vi "Barrier for IV curve.vi"() -> ()   [LabVIEW 2016]
panel:
  out "Barrier average 2":dbl=0.21135603486952198 format="%#_6p"
  out "Barrier for backward IV 2":dbl=0.22242669607101634 format="%#_6p"
  out "Barrier for forward IV 2":dbl=0.20028537366802762 format="%#_6p"
  out "IV after extracting current offset at zero bias":cluster{"Time Stamps":dbl[], dbl[]}[](graph)
  out "IV after extracting current offset at zero bias":cluster{"Time Stamps":dbl[], "Y":dbl[]}(graph)
  out "Backward offset":dbl=1.766897762857724e-08 format="%#_6p"
  out "Forward offset":dbl=-1.6472324480187406e-08 format="%#_6p"
  out "size(s)":i32=525
  out "IV without extracting current offset at zero bias":cluster{"Time Stamps":dbl[], "Y":dbl[]}[](graph)
  out "Barrier average":dbl=0.28652409507268245 format="%#_6p"
  out "Barrier for forward IV":dbl=0.24381885922702945 format="%#_6p"
  out "Barrier for backward IV":dbl=0.32922933091833545 format="%#_6p"
  in  "Linear fitting step":i32=32
  out "min index(es)":i32=394 format="%.0p"
  out "min value":dbl=-0.49999890379533224 format="%#_6p"
  out "max index(es)":i32=131 format="%.0p"
  out "max value":dbl=0.49999729304706686 format="%#_6p"
  in  "Input IV curve":cluster{"Time Stamps":dbl[], "Y":dbl[]}(graph)={"Time Stamps"=array[525 elements], "Y"=array[525 elements]}
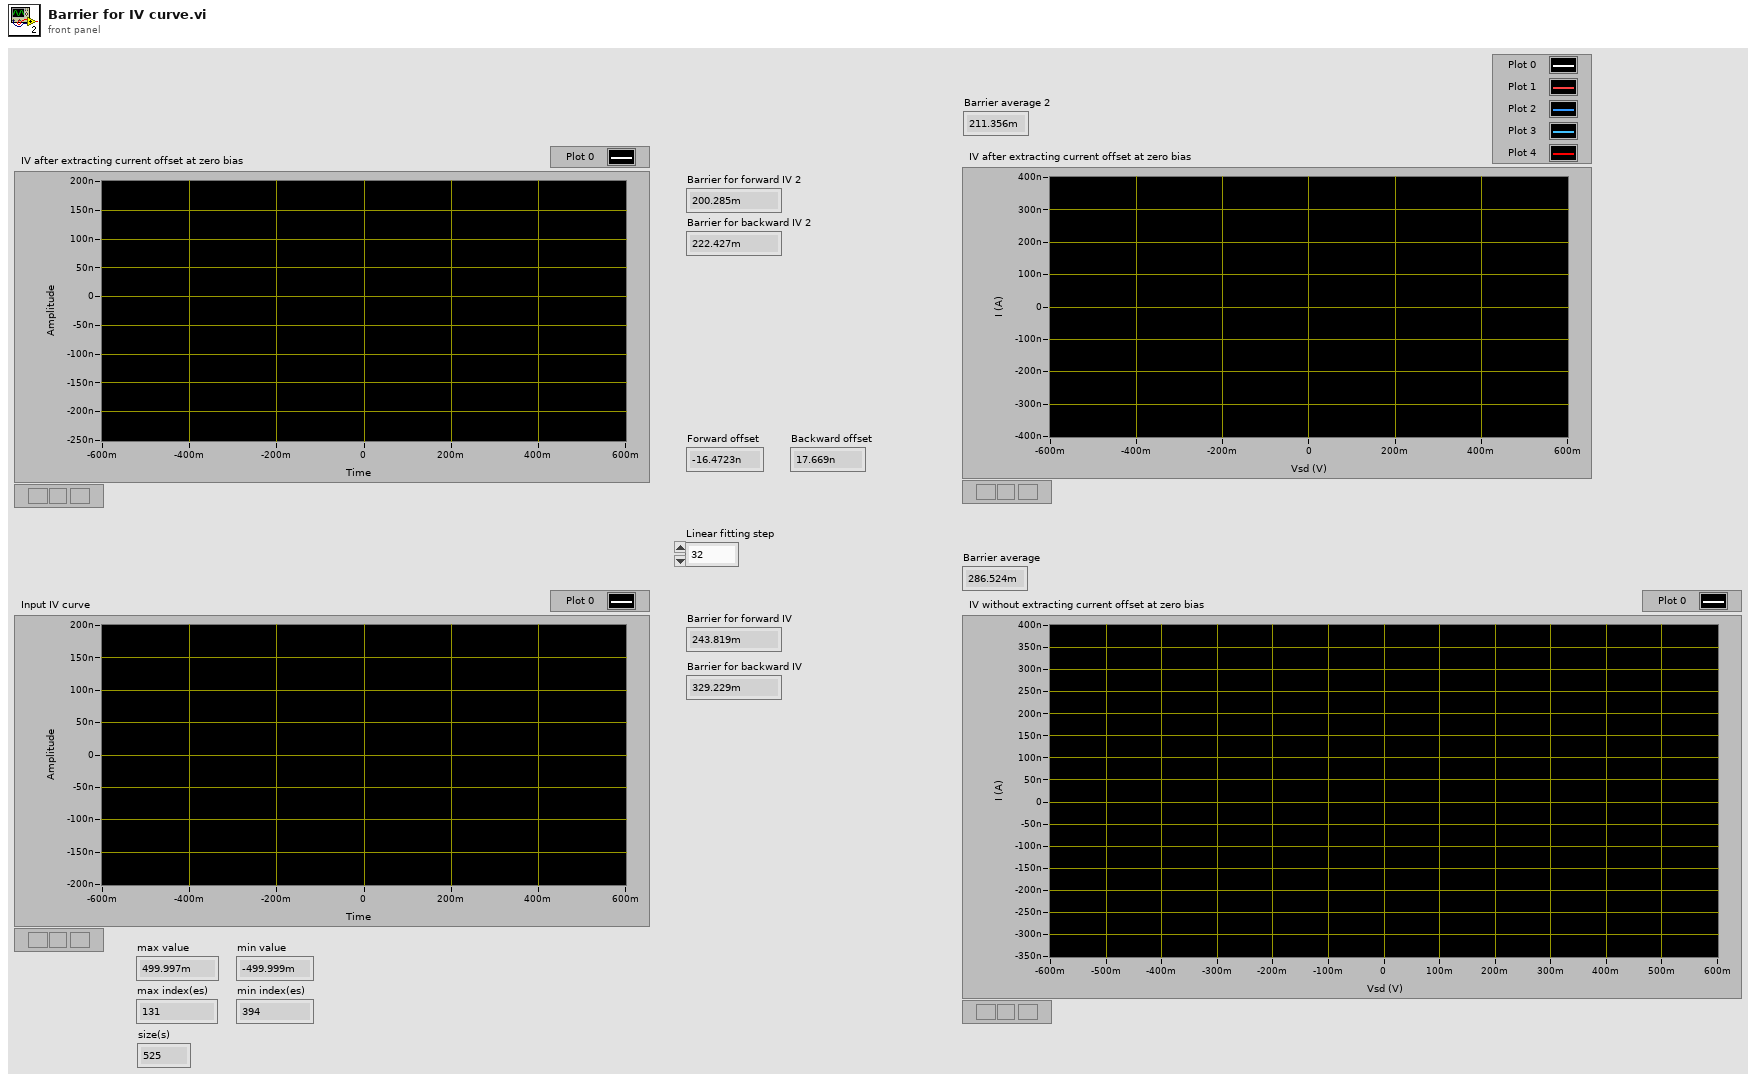
[diagram p1: front panel]
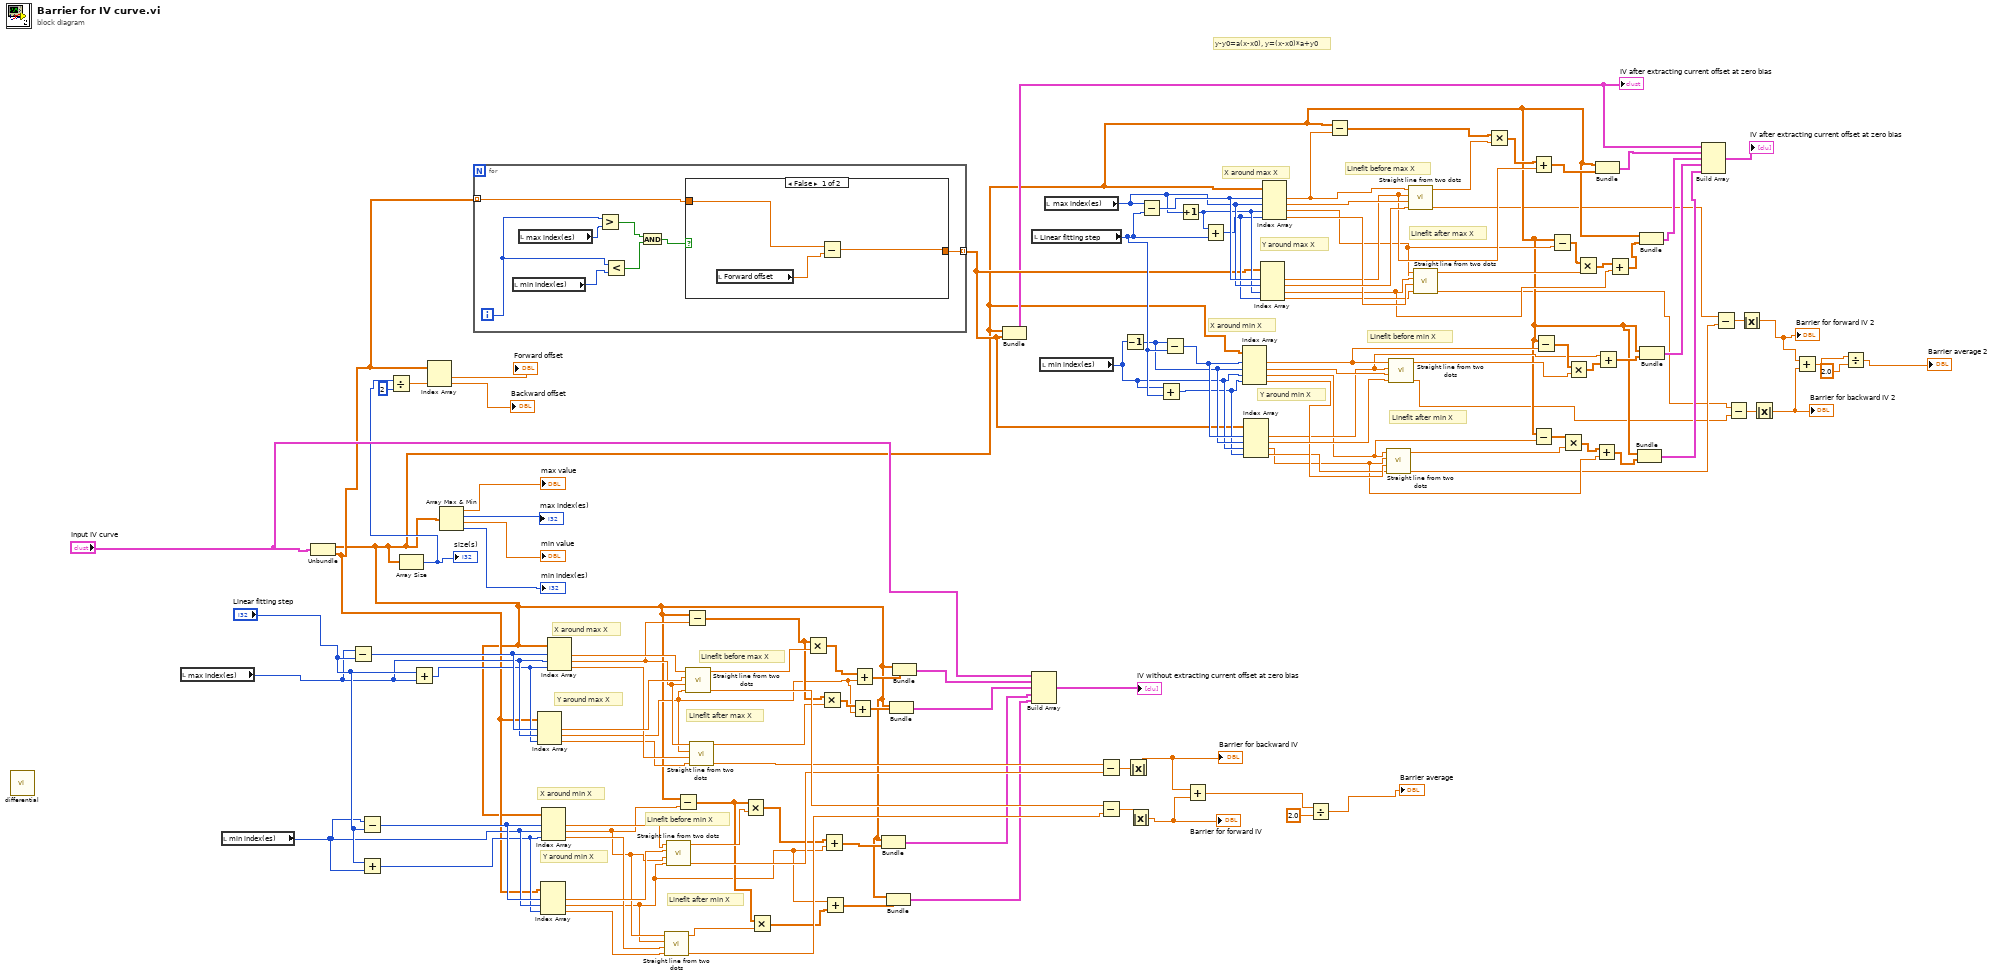
[diagram p0: block diagram]
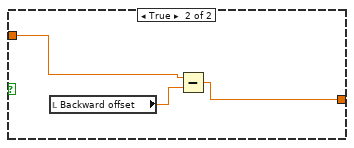
[diagram p2: hidden frame]
diagram:
  # "y-y0=a(x-x0), y=(x-x0)*a+y0"
  # "Linefit after min X"
  # "Linefit before min X"
  # "Linefit after max X"
  # "Linefit before max X"
  # "Y around min X"
  # "X around min X"
  # "Y around max X"
  # "X around max X"
  # "Linefit after min X"
  # "Linefit before min X"
  # "Linefit after max X"
  # "Linefit before max X"
  # "Y around min X"
  # "X around min X"
  # "Y around max X"
  # "X around max X"
  n1 = call <userlib>:"differential.vi"() -> ()  [unwired: 4 in, 1 out]
  n2 = local read "max index(es)"() -> (w113:i32)
  n3 = local read "min index(es)"() -> (w107:i32)
  n4 = Unbundle("Input IV curve") -> ("Time Stamps"=w13:dbl[], "Y"=w61:dbl[])
  n5 = Subtract(x=w113, y="Linear fitting step") -> (x-y=w114:i32)
  n6 = Subtract(x=w107, y="Linear fitting step") -> (x-y=w108:i32)
  n7 = Add(x="Linear fitting step", y=w107) -> (x+y=w106:i32)
  n8 = Array Size(array=w13) -> (size(s)=w63:i32)
  "size(s)" <- w63
  n9 = Divide(x=w63, y=2) -> (x/y=w66:dbl)
  n10 = Add(x="Linear fitting step", y=w113) -> (x+y=w112:i32)
  n11 = Index Array(array=w61, index #2=w66) -> (element #1=→"Forward offset":dbl, element #2=→"Backward offset":dbl)  [unwired: 1 in]
  n12 = Array Max & Min(array=w13) -> (max value=→"max value":dbl, max index (indices)=→"max index(es)":i32, min value=→"min value":dbl, min index (indices)=→"min index(es)":i32)
  n13 = for {
    tunnel: w61 -> [w122] mode=indexing
    tunnel: [w121] -> w51 mode=indexing
    i -> [w127]
    n14 = local read "min index(es)"() -> (w126:i32)
    n15 = local read "max index(es)"() -> (w128:i32)
    n16 = Greater?(x=w127, y=w128) -> (0:w125:bool)
    n17 = Less?(x=w127, y=w126) -> (x < y?=w124:bool)
    n18 = And(x=w125, y=w124) -> (x .and. y?=w123:bool)
    n19 = case shown="False" w123 {
      tunnel: w122 -> [w131 w134]
      tunnel: [w129 w132] -> w121
      frame False {
        n20 = local read "Forward offset"() -> (w130:dbl)
        n21 = Subtract(x=w131, y=w130) -> (x-y=w129:dbl)
      }
      frame True {
        n22 = local read "Backward offset"() -> (w133:dbl)
        n23 = Subtract(x=w134, y=w133) -> (x-y=w132:dbl)
      }
    }
  }
  n24 = Index Array(array=w61, index #1=w114, index #2=w113, index #3=w112) -> (element #1=w111:dbl, element #2=w80:dbl, element #3=w109:dbl)
  n25 = Index Array(array=w61, index #1=w108, index #2=w107, index #3=w106) -> (element #1=w104:dbl, element #2=w71:dbl, element #3=w102:dbl)
  n26 = Index Array(array=w13, index #1=w108, index #2=w107, index #3=w106) -> (element #1=w105:dbl, element #2=w77:dbl, element #3=w103:dbl)
  n27 = Index Array(array=w13, index #1=w114, index #2=w113, index #3=w112) -> (element #1=w115:dbl, element #2=w90:dbl, element #3=w110:dbl)
  n28 = call "Straight line from two dots.vi"("Y2"=w102, "X2"=w103, "Y1"=w71, "X1"=w77) -> ("X intercept"=w100:dbl, "Slope"=w72:dbl)  [unwired: 6 in]
  n29 = call "Straight line from two dots.vi"("Y2"=w71, "X2"=w77, "Y1"=w104, "X1"=w105) -> ("X intercept"=w98:dbl, "Slope"=w76:dbl)  [unwired: 6 in]
  n30 = Subtract(x=w13, y=w77) -> (x-y=w73:dbl[])
  n31 = Subtract(x=w13, y=w90) -> (x-y=w82:dbl[])
  n32 = call "Straight line from two dots.vi"("Y2"=w80, "X2"=w90, "Y1"=w111, "X1"=w115) -> ("X intercept"=w101:dbl, "Slope"=w89:dbl)  [unwired: 6 in]
  n33 = call "Straight line from two dots.vi"("Y2"=w109, "X2"=w110, "Y1"=w80, "X1"=w90) -> ("X intercept"=w99:dbl, "Slope"=w83:dbl)  [unwired: 6 in]
  n34 = Multiply(x=w73, y=w76) -> (x*y=w75:dbl[])
  n35 = Multiply(x=w73, y=w72) -> (x*y=w70:dbl[])
  n36 = Multiply(x=w82, y=w89) -> (x*y=w88:dbl[])
  n37 = Multiply(x=w82, y=w83) -> (x*y=w81:dbl[])
  n38 = Add(x=w75, y=w71) -> (x+y=w74:dbl[])
  n39 = Add(x=w71, y=w70) -> (x+y=w69:dbl[])
  n40 = Add(x=w81, y=w80) -> (x+y=w79:dbl[])
  n41 = Add(x=w88, y=w80) -> (x+y=w87:dbl[])
  n42 = Bundle("Time Stamps"=w13, w74) -> (w68:cluster{"Time Stamps":dbl[], dbl[]})  [unwired: 1 in]
  n43 = Bundle("Time Stamps"=w13, w69) -> (w67:cluster{"Time Stamps":dbl[], dbl[]})  [unwired: 1 in]
  n44 = Bundle("Time Stamps"=w13, w79) -> (w78:cluster{"Time Stamps":dbl[], dbl[]})  [unwired: 1 in]
  n45 = Bundle("Time Stamps"=w13, w87) -> (w85:cluster{"Time Stamps":dbl[], dbl[]})  [unwired: 1 in]
  n46 = Bundle("Time Stamps"=w13, w51) -> (w36:cluster{"Time Stamps":dbl[], dbl[]})  [unwired: 1 in]
  "IV after extracting current offset at zero bias" <- w36
  n47 = local read "Linear fitting step"() -> (w56:i32)
  n48 = Build Array("Input IV curve", w85, w78, w68, w67) -> (→"IV without extracting current offset at zero bias":cluster{"Time Stamps":dbl[], "Y":dbl[]}[])
  n49 = local read "min index(es)"() -> (w53:i32)
  n50 = local read "max index(es)"() -> (w59:i32)
  n51 = Subtract(x=w99, y=w98) -> (x-y=w97:dbl)
  n52 = Subtract(x=w101, y=w100) -> (x-y=w96:dbl)
  n53 = Decrement(x=w53) -> (x-1=w54:i32)
  n54 = Absolute Value(x=w97) -> (abs(x)=w95:dbl)
  "Barrier for backward IV" <- w95
  n55 = Absolute Value(x=w96) -> (abs(x)=w94:dbl)
  "Barrier for forward IV" <- w94
  n56 = Subtract(x=w59, y=w56) -> (x-y=w60:i32)
  n57 = Add(x=w53, y=w56) -> (x+y=w52:i32)
  n58 = Subtract(x=w54, y=w56) -> (x-y=w55:i32)
  n59 = Increment(x=w59) -> (x+1=w58:i32)
  n60 = Add(x=w95, y=w94) -> (x+y=w93:dbl)
  n61 = Add(x=w58, y=w56) -> (x+y=w57:i32)
  n62 = Index Array(array=w13, index #1=w55, index #2=w54, index #3=w53, index #4=w52) -> (element #1=w26:dbl, element #2=w46:dbl, element #3=w19:dbl, element #4=w44:dbl)
  n63 = Index Array(array=w51, index #1=w55, index #2=w54, index #3=w53, index #4=w52) -> (element #1=w23:dbl, element #2=w45:dbl, element #3=w16:dbl, element #4=w43:dbl)
  n64 = Index Array(array=w51, index #1=w60, index #2=w59, index #3=w58, index #4=w57) -> (element #1=w38:dbl, element #2=w49:dbl, element #3=w29:dbl, element #4=w47:dbl)
  n65 = Index Array(array=w13, index #1=w60, index #2=w59, index #3=w58, index #4=w57) -> (element #1=w42:dbl, element #2=w50:dbl, element #3=w33:dbl, element #4=w48:dbl)
  n66 = Divide(x=w93, y=2.0) -> (x/y=→"Barrier average":dbl)
  n67 = Subtract(x=w13, y=w42) -> (x-y=w41:dbl[])
  n68 = call "Straight line from two dots.vi"("Y2"=w43, "X2"=w44, "Y1"=w16, "X1"=w19) -> ("X intercept"=w10:dbl, "Slope"=w17:dbl)  [unwired: 6 in]
  n69 = call "Straight line from two dots.vi"("Y2"=w45, "X2"=w46, "Y1"=w23, "X1"=w26) -> ("X intercept"=w7:dbl, "Slope"=w24:dbl)  [unwired: 6 in]
  n70 = call "Straight line from two dots.vi"("Y2"=w49, "X2"=w50, "Y1"=w38, "X1"=w42) -> ("X intercept"=w11:dbl, "Slope"=w40:dbl)  [unwired: 6 in]
  n71 = call "Straight line from two dots.vi"("Y2"=w47, "X2"=w48, "Y1"=w29, "X1"=w33) -> ("X intercept"=w8:dbl, "Slope"=w31:dbl)  [unwired: 6 in]
  n72 = Multiply(x=w41, y=w40) -> (x*y=w39:dbl[])
  n73 = Add(x=w39, y=w38) -> (x+y=w37:dbl[])
  n74 = Subtract(x=w13, y=w19) -> (x-y=w18:dbl[])
  n75 = Subtract(x=w13, y=w26) -> (x-y=w25:dbl[])
  n76 = Subtract(x=w13, y=w33) -> (x-y=w32:dbl[])
  n77 = Multiply(x=w18, y=w17) -> (x*y=w15:dbl[])
  n78 = Multiply(x=w25, y=w24) -> (x*y=w22:dbl[])
  n79 = Multiply(x=w32, y=w31) -> (x*y=w30:dbl[])
  n80 = Add(x=w15, y=w16) -> (x+y=w14:dbl[])
  n81 = Bundle("Time Stamps"=w13, w37) -> (w35:cluster{"Time Stamps":dbl[], dbl[]})  [unwired: 1 in]
  n82 = Add(x=w23, y=w22) -> (x+y=w21:dbl[])
  n83 = Add(x=w30, y=w29) -> (x+y=w28:dbl[])
  n84 = Bundle("Time Stamps"=w13, w14) -> (w12:cluster{"Time Stamps":dbl[], dbl[]})  [unwired: 1 in]
  n85 = Bundle("Time Stamps"=w13, w28) -> (w27:cluster{"Time Stamps":dbl[], dbl[]})  [unwired: 1 in]
  n86 = Bundle("Time Stamps"=w13, w21) -> (w20:cluster{"Time Stamps":dbl[], dbl[]})  [unwired: 1 in]
  n87 = Build Array(w36, w35, w27, w20, w12) -> (→"IV after extracting current offset at zero bias":cluster{"Time Stamps":dbl[], dbl[]}[])
  n88 = Subtract(x=w11, y=w10) -> (x-y=w9:dbl)
  n89 = Subtract(x=w8, y=w7) -> (x-y=w6:dbl)
  n90 = Absolute Value(x=w9) -> (abs(x)=w5:dbl)
  "Barrier for forward IV 2" <- w5
  n91 = Absolute Value(x=w6) -> (abs(x)=w3:dbl)
  "Barrier for backward IV 2" <- w3
  n92 = Add(x=w5, y=w3) -> (x+y=w2:dbl)
  n93 = Divide(x=w2, y=2.0) -> (x/y=→"Barrier average 2":dbl)
